vi "Task Type.vi"(11 "ChartGuiTask in":refnum<class "ChartGuiTask.lvclass">) -> (2 "Task Type":string)   [LabVIEW 2020, in "VolatusDemo.lvlib" / "ChartGuiTask.lvclass"]
uses:
  ChartGuiTask.lvclass
  ChartGuiTask.lvclass/ChartGuiTask.ctl
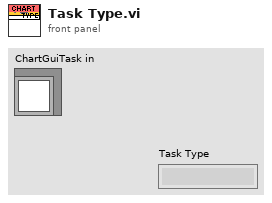
[diagram p1: front panel]
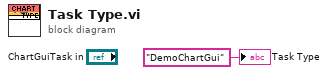
[diagram p0: block diagram]
diagram:
  "Task Type" <- "DemoChartGui" ("Task Type")
